vi "ProcessLidarData.vi"(0 "WhatAroundMe?MM":cluster{"T":dbl, "Range":dbl, "Bearing":dbl}[](array[cluster])) -> (1 "Collision":bool, 2 "data array [mag, phase (deg)]":cluster{"magnitude":dbl, "phase":dbl}[](array[cluster]))   [LabVIEW 2010]
doc: "Strips time cell out of LIDAR array data"
panel:
  # "This subVI just strips off \nthe time data so that \nLIDAR data can be polar \nplotted."
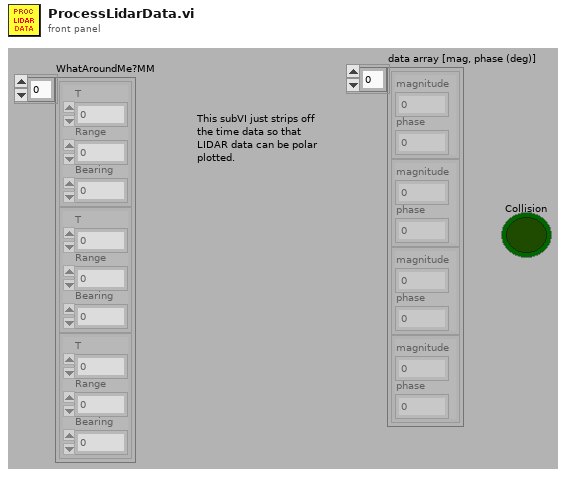
[diagram p1: front panel]
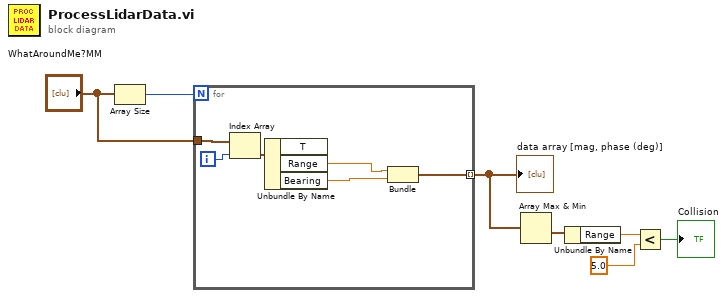
[diagram p0: block diagram]
diagram:
  n1 = Array Size(array="WhatAroundMe?MM") -> (size(s)=w7:i32)
  n2 = for {
    N: w7 -> [_]
    tunnel: "WhatAroundMe?MM" -> [w13]
    tunnel: [w8] -> w5 mode=indexing
    i -> [w12]
    n3 = Index Array "Index Array"(array=w13, index=w12) -> (element=w11:cluster{"T":dbl, "Range":dbl, "Bearing":dbl})
    n4 = Unbundle By Name "Unbundle By Name"(w11) -> ("Range"=w10:dbl, "Bearing"=w9:dbl)  [unwired: 1 out]
    n5 = Bundle "Bundle"("Range"=w10, "Bearing"=w9) -> (w8:cluster{"Range":dbl, "Bearing":dbl})  [unwired: 1 in]
  }
  "data array [mag, phase (deg)]" <- w5
  n6 = Array Max & Min(array=w5) -> (min value=w4:cluster{"Range":dbl, "Bearing":dbl})  [unwired: 3 out]
  n7 = Unbundle By Name(w4) -> ("Range"=w3:dbl)
  n8 = Less?(x=w3, y=5.0) -> (x < y?=→"Collision":bool)
